vi "PSRR.vi"() -> ()   [LabVIEW 2020]
doc: "For every time interval of n second, where n is the Wait Time in seconds (not less than 2 seconds), the VI will call Synchronous PSRR.vi. If there are no errors, the obtained data will be plotted in a chart.\n\n1. Error Log - If Error Log is enabled, log entry into the Error Log Table (for both error and warning).\n2. Last Error Details – will be updated with the details of Last Error or Warning that happened.\n3. Error? - In case of an error, Error? LED will be ON until the error is cleared."
uses:
  Typedef/QueueOperation.ctl
  Typedef/State & Varaint.ctl
  Typedef/LV2_User_Event.ctl
  Typedef/Data Cluster.ctl
  Typedef/Timer_Cluster.ctl
  Typedef/LED_Colour.ctl
  <vilib>/Utility/miscctls.llb/LVRowAndColumnUnsignedTypeDef.ctl
panel:
  out "Error?":bool
  in  "Error Log":bool
  out "Error Log Table":string[][](table)
  in  "Exit":bool
  out "Time":string
  in  "Wait Time (sec)":i32=2 min=2
  out "Waveform Chart":i32(graph)
  out "Error Code":string
  out "Type":string
  out "Description":string
  out "Error Out":errorcluster
  out "Last Read PSRR (dB)":i32
  in  "Error In":errorcluster
  # "PSRR"
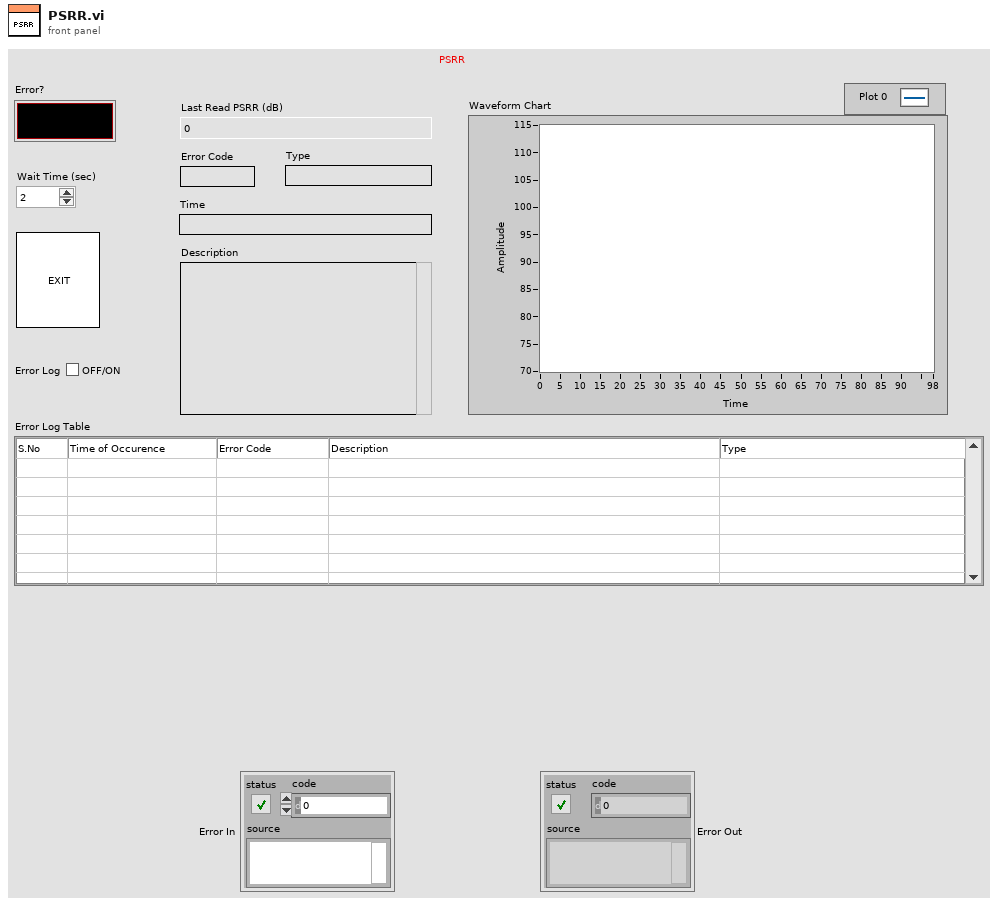
[diagram p1: front panel]
types:
  T1 = typedef "QueueOperation.ctl" = enum16{"Create", "Enqueue 1", "Enqueue N", "Enstack 1", "Enstack N", "Dequeue", "Flush", "Release"}
  T2 = typedef "LV2_User_Event.ctl" = enum16{"Create", "Generate", "Read", "Destroy"}
  T3 = typedef "State & Varaint.ctl" = cluster{"State":string, "Variant":variant}
  T4 = typedef "LVRowAndColumnUnsignedTypeDef.ctl" = cluster{"Row":u32, "Column":u32}
  T5 = typedef "Data Cluster.ctl" = cluster{"Exit":bool, "Error Log":bool, "Wait Time (sec)":i32, "Last Read PSRR (dB)":i32, "Waveform Chart":i32, "Error Code":string, "Type":string, "Time":string, "Description":string, "Error?":bool, "Error Info":errorcluster, "Timer":T6, "Passive Error Counter":i32, "Unknown Error Counter":i32, "Serial Number":i32, "Error Logging string array":string[][], "Popup Message":string, "Autoscroll":u32, "LED cluster":T7}
  T6 = typedef "Timer_Cluster.ctl" = cluster{"Previous":dbl, "Set Time":dbl, "Start":bool, "Elapsed":dbl}
  T7 = typedef "LED_Colour.ctl" = cluster{"Boolean Text":string, "Colors":cluster{u32, u32}[], "Txt Color":u32}
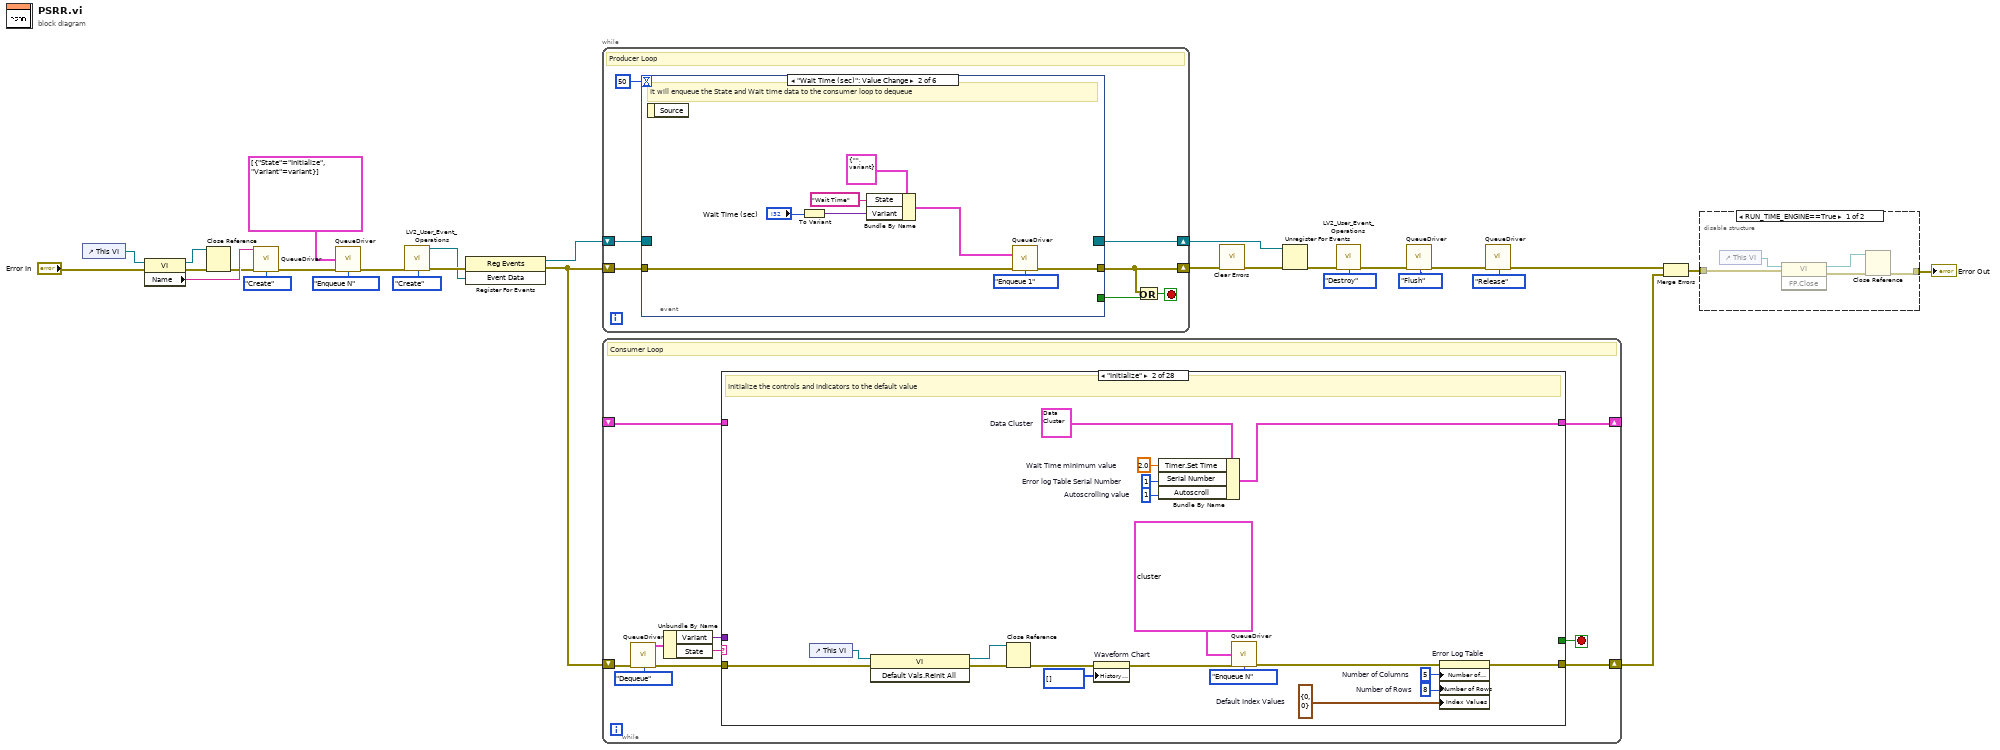
[diagram p0: block diagram]
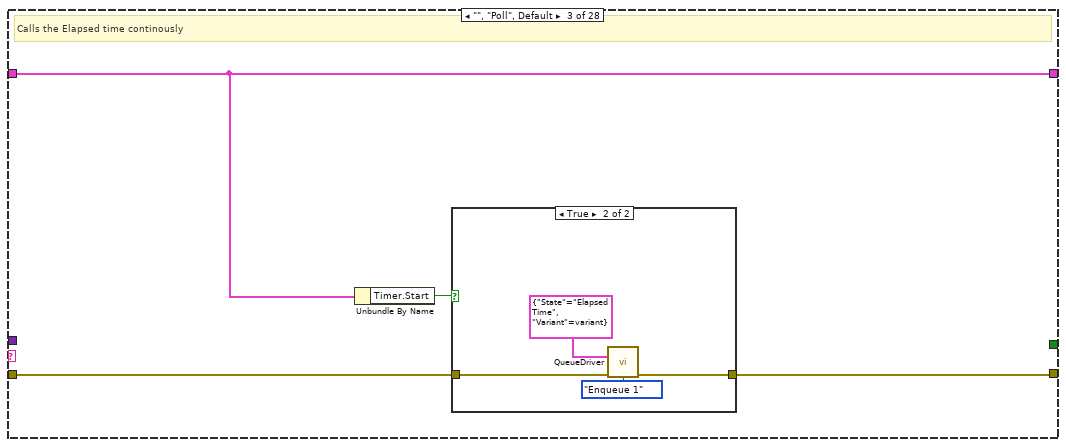
[diagram p4: hidden frame]
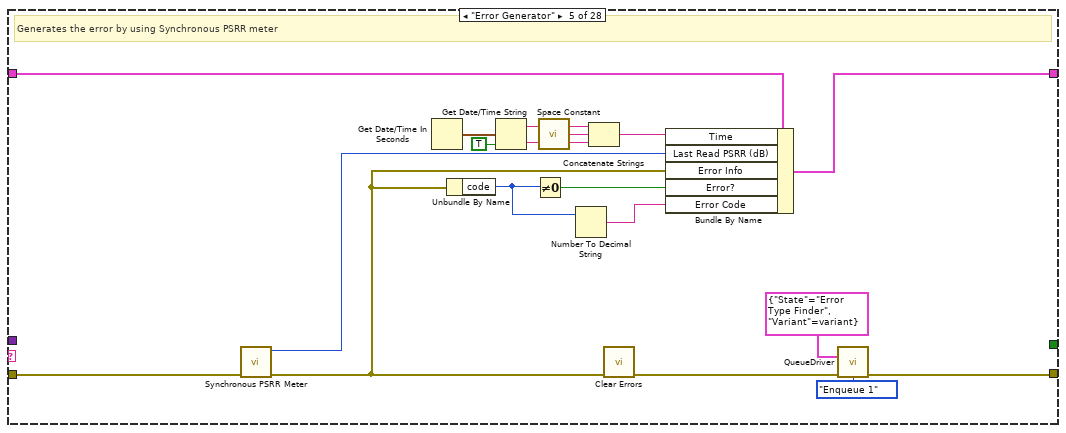
[diagram p7: hidden frame]
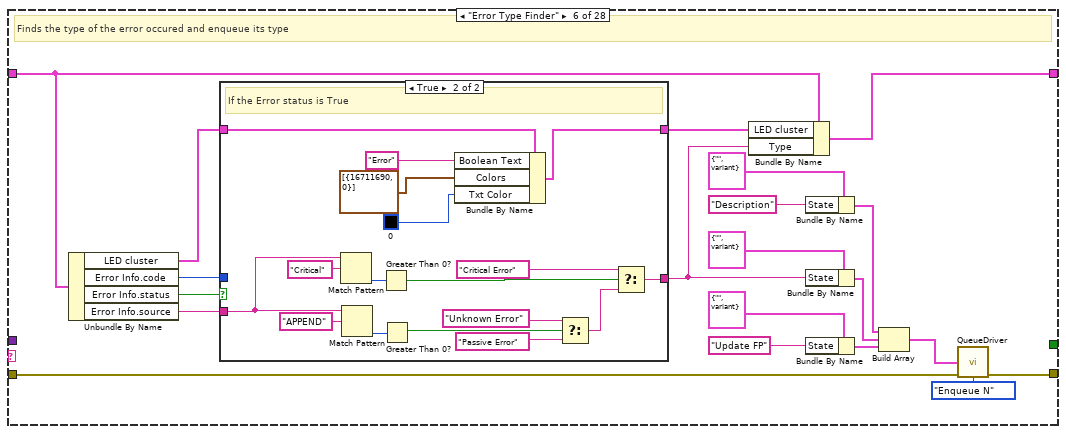
[diagram p8: hidden frame]
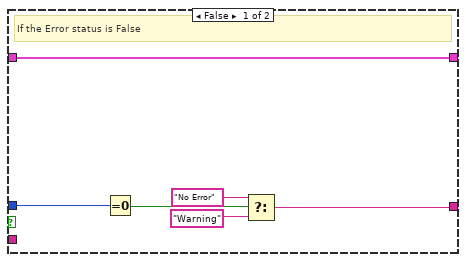
[diagram p9: hidden frame]
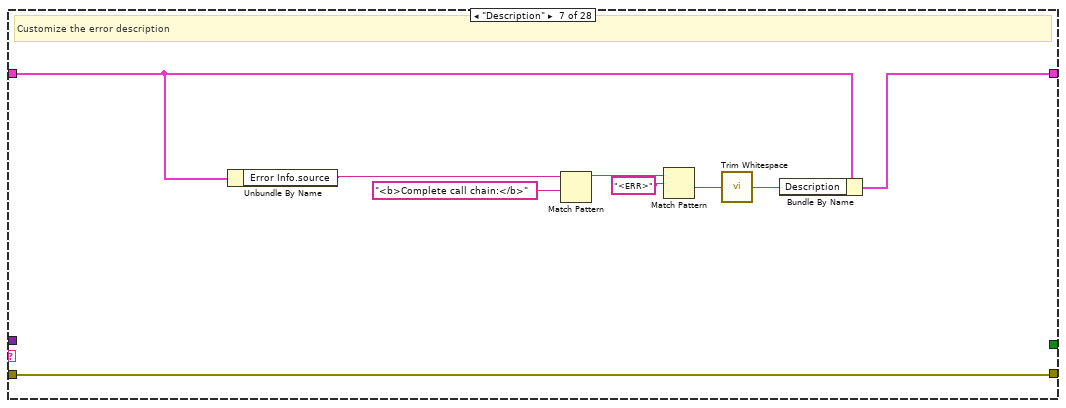
[diagram p10: hidden frame]
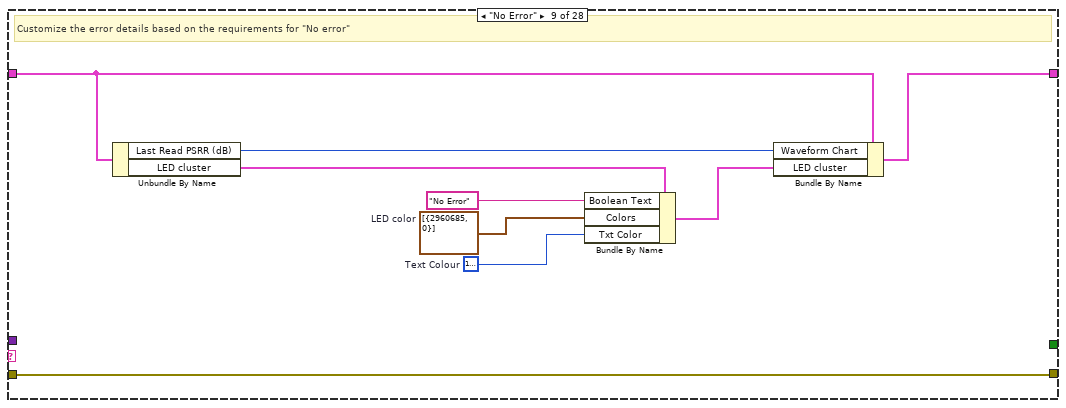
[diagram p12: hidden frame]
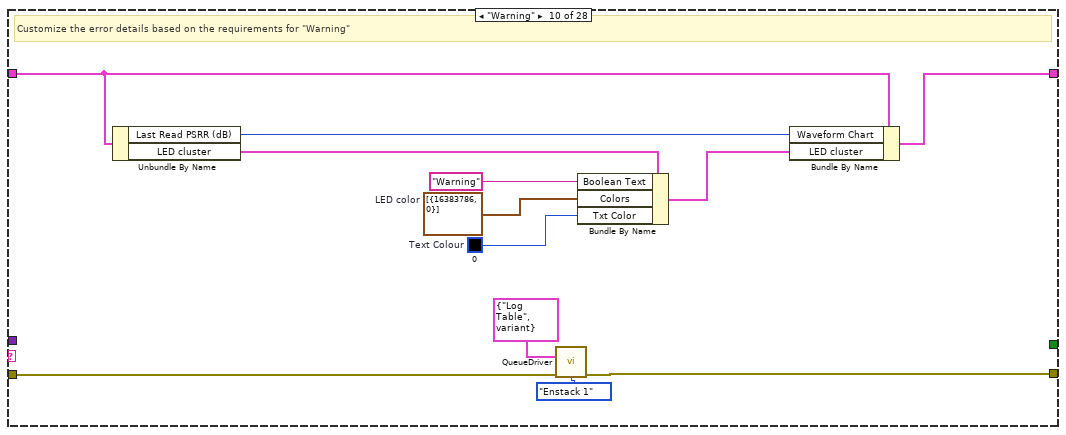
[diagram p13: hidden frame]
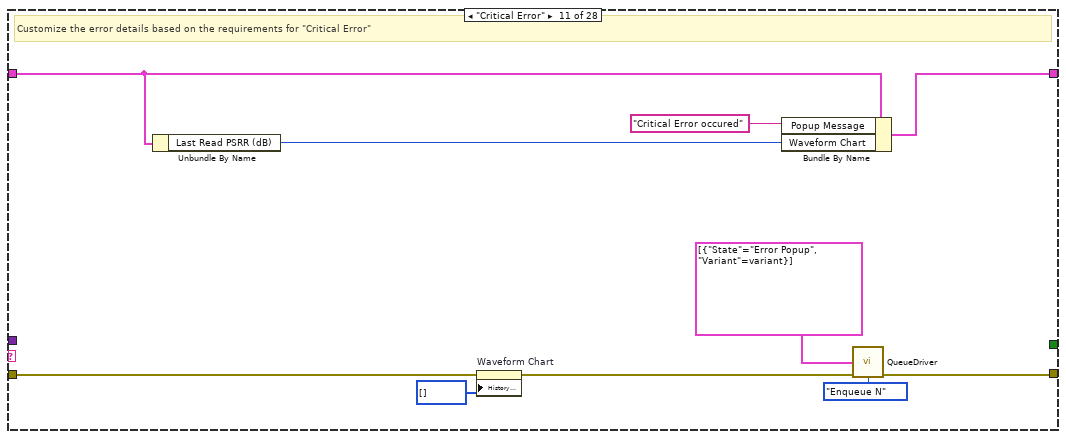
[diagram p14: hidden frame]
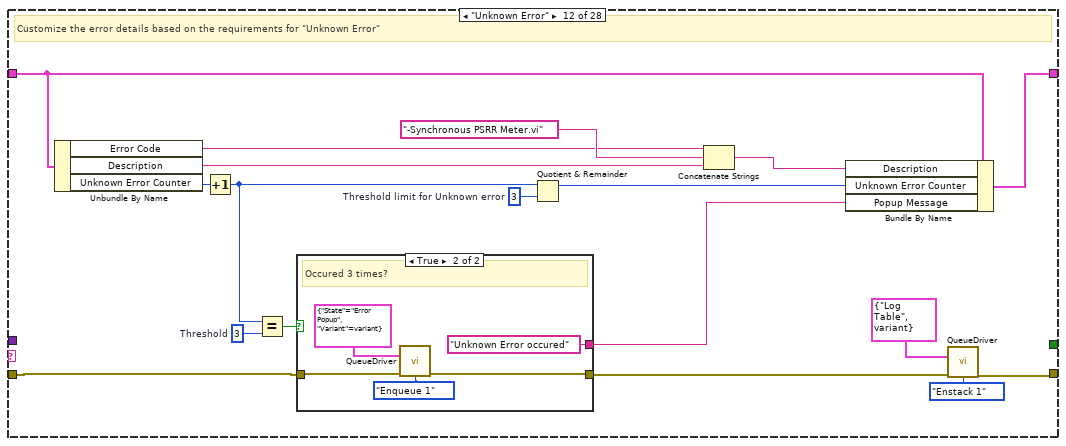
[diagram p15: hidden frame]
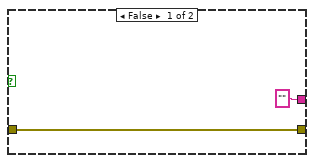
[diagram p16: hidden frame]
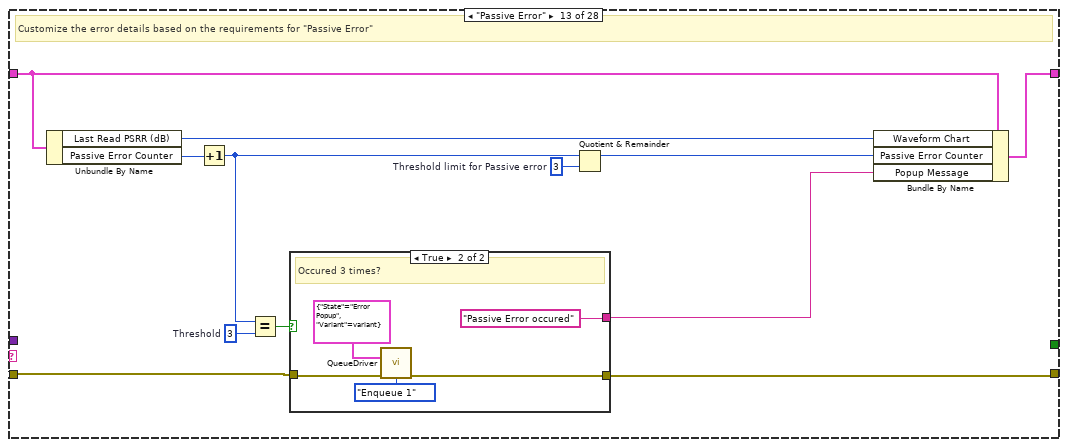
[diagram p17: hidden frame]
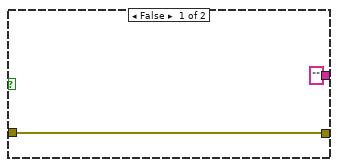
[diagram p18: hidden frame]
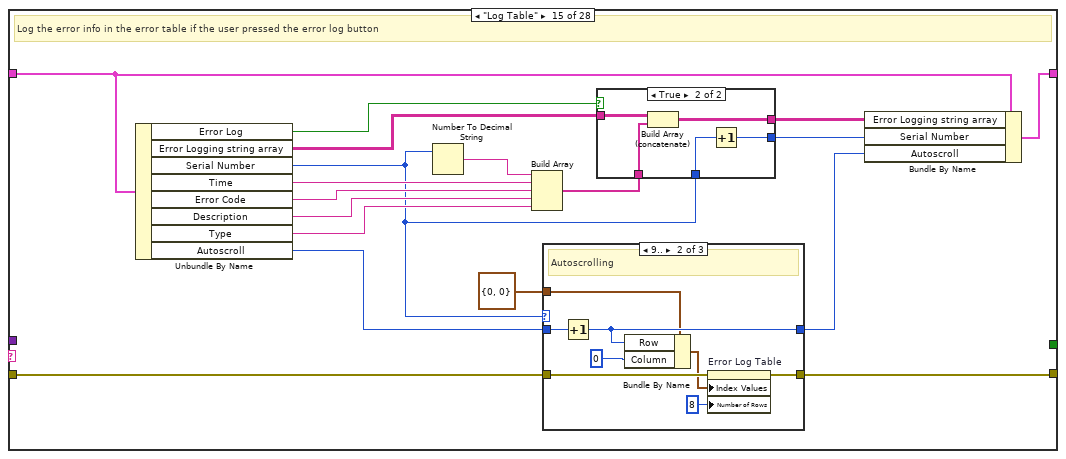
[diagram p20: hidden frame]
diagram:
  n1 = control-ref of="This VI"() -> (w6:refnum<vi>)
  n2 = property class="VI"(reference=w6, error in="Error In") -> (reference out=w3:refnum<vi>, error out=w5:errorcluster, "Name"=w27:string)
  n3 = Close Reference(reference=w3, error in (no error)=w5) -> (error out=w4:errorcluster)
  n4 = call "QueueDriver.vi"("Queue Name"=w27, "Error in (no error)"=w4, "Operations"=QueueOperation."Create") -> ("Error out"=w26:errorcluster)  [unwired: 11 in, 1 out]
  n5 = call "QueueDriver.vi"("Array of States & Data"=T3[] [{"State"="Initialize", "Variant"=variant}], "Error in (no error)"=w26, "Operations"=QueueOperation."Enqueue N") -> ("Error out"=w23:errorcluster)  [unwired: 11 in, 1 out]
  n6 = call "LV2_User_Event_Operations.vi"("Error In"=w23, "Operation"=LV2_User_Event."Create") -> ("Event Data"=w19:refnum<user-event>, "Error Out"=w21:errorcluster)  [unwired: 12 in]
  n7 = register-events(error in=w21, w19) -> (reference out=w18:refnum<event-registration>, error out=w20:errorcluster)  [unwired: 1 in]
  n8 = while {
    shift-right: [w30] -> w16
    shift-left: w20 -> [w35]
    shift-right: [w33] -> w14
    shift-left: w18 -> [w34]
    stop <- w32 stop-if-true
    # "Producer Loop"
    n9 = event shown="[1] \"Wait Time (sec)\": Value Change" {
      selector: w34 -> [_ _ _ _ _ _]
      dyn-events: [_ _ _ _ _ _] -> w33
      timeout: 50 -> [_ _ _ _ _ _]
      tunnel: [w37 w38 w52 w54 w58 w64] -> w30
      tunnel: w35 -> [w37 w45 w53 w54 w59 w65]
      tunnel: [_ _ _ TRUE w60 TRUE] -> w31
      event Timeout {
        # "This block executes when there is no event triggered"
        n10 = event-data() -> ()  [unwired: 1 in, 1 out]
      }
      event "Wait Time (sec)": Value Change {
        # "It will enqueue the State and Wait time data to the consumer loop to dequeue"
        n11 = event-data() -> ()  [unwired: 1 in, 1 out]
        n12 = To Variant(anything="Wait Time (sec)") -> (Variant=w40:variant)
        n13 = Bundle By Name(cluster=T3 {"State"="", "Variant"=variant} ("State & Data"), "State"="Wait Time", "Variant"=w40) -> (w39:T3)
        n14 = call "QueueDriver.vi"("State & Data"=w39, "Error in (no error)"=w45, "Operations"=QueueOperation."Enqueue 1") -> ("Error out"=w38:errorcluster)  [unwired: 11 in, 1 out]
      }
      event "Error Log": Value Change {
        # "It will enqueue the State and Error Log data to the consumer loop to dequeue"
        n15 = event-data() -> ()  [unwired: 1 in, 1 out]
        n16 = To Variant(anything="Error Log") -> (Variant=w48:variant)
        n17 = Bundle By Name(cluster=T3 {"State"="", "Variant"=variant} ("State & Data"), "State"="Error Log", "Variant"=w48) -> (w47:T3)
        n18 = call "QueueDriver.vi"("State & Data"=w47, "Error in (no error)"=w53, "Operations"=QueueOperation."Enqueue 1") -> ("Error out"=w52:errorcluster)  [unwired: 11 in, 1 out]
      }
      event User Event {
        # "Stops the producer loop when consumer loop generates the user event"
        n19 = event-data() -> ()  [unwired: 1 in, 1 out]
      }
      event Panel Close? {
        w60 = TRUE
        # "Stops the VI when the panel close button is pressed"
        n20 = event-data() -> ()  [unwired: 1 in, 1 out]
        n21 = call "QueueDriver.vi"("State & Data"=T3 {"State"="Exit", "Variant"=variant}, "Error in (no error)"=w59, "Operations"=QueueOperation."Enstack 1") -> ("Error out"=w58:errorcluster)  [unwired: 11 in, 1 out]
        n22 = event-data("Discard?"=w60) -> ()  [unwired: 1 in, 1 out]
      }
      event "Exit": Value Change {
        # "Stops the VI when the exit button is pressed"
        n23 = event-data() -> ()  [unwired: 1 in, 1 out]
        n24 = call "QueueDriver.vi"("State & Data"=T3 {"State"="Exit", "Variant"=variant}, "Error in (no error)"=w65, "Operations"=QueueOperation."Enstack 1") -> ("Error out"=w64:errorcluster)  [unwired: 11 in, 1 out]
      }
    }
    n25 = Or(x=w30, y=w31) -> (x .or. y?=w32:bool)
  }
  n26 = while {
    shift-right: [w69] -> w13
    shift-left: w20 -> [w75]
    shift-right: [w68] -> _
    shift-left: _ -> [w67]
    stop <- w66 stop-if-true
    # "Consumer Loop"
    n27 = call "QueueDriver.vi"("Error in (no error)"=w75, "Operations"=QueueOperation."Dequeue") -> ("Dequeued State & Variant"=w73:T3, "Error out"=w70:errorcluster)  [unwired: 12 in]
    n28 = Unbundle By Name(w73) -> ("Variant"=w71:variant, "State"=w72:string)
    n29 = case shown="\"Initialize\"" w72 {
      tunnel: w71 -> [_ _ _ _ _ _ _ _ _ _ _ _ _ _ _ _ _ _ w337 w345 _ _ _ _ _ _ _ _]
      tunnel: w70 -> [w76 w96 w100 w107 w125 w142 w169 w179 w185 w196 w202 w215 w236 w256 w263 w304 w318 w332 w339 w346 w348 w350 w359 w371 w379 w384 w400 w401]
      tunnel: [w76 w84 w99 w107 w121 w141 w169 w179 w185 w197 w206 w225 w238 w256 w264 w305 w317 w332 w334 w343 w348 w350 w359 w370 w379 w381 w400 w404] -> w69
      tunnel: [w77 w92 w97 w106 w123 w143 w176 w178 w187 w199 w209 w226 w246 w255 w273 w307 w322 w331 w333 w342 w347 w354 w358 w368 w378 w383 w399 w405] -> w68
      tunnel: w67 -> [w77 _ w97 w106 w124 w144 w177 w178 w188 w200 w210 w228 w247 w255 w274 w307 w322 w331 w336 w344 w347 w355 w360 w369 w378 w383 w399 w405]
      tunnel: [_ _ _ _ _ _ _ _ _ _ _ _ _ _ _ _ _ _ _ _ _ _ _ _ _ w380 _ TRUE] -> w66
      frame "/*******Initialize the VI*******/" {
      }
      frame "Initialize" {
        w81 = T4 {"Row"=0, "Column"=0}  # Default Index Values
        w82 = u32 8  # Number of Rows
        w83 = u32 5  # Number of Columns
        w86 = u32 1  # Autoscrolling value
        w90 = 1  # Error log Table Serial Number
        w91 = 2.0  # Wait Time minimum value
        w94 = T5 {"Exit"=FALSE, "Error Log"=FALSE, "Wait Time (sec)"=0, "Last Read PSRR (dB)"=0, "Waveform Chart"=0, "Error Code"="", "Type"="", "Time"="", "Description"="", "Error?"=FALSE, "Error Info"={"status"=FALSE, "code"=0, "source"=""}, "Timer"={"Previous"=0.0, "Set Time"=0.0, "Start"=FALSE, "Elapsed"=0.0}, "Passive Error Counter"=0, "Unknown Error Counter"=0, "Serial Number"=0, "Error Logging string array"=[], "Popup Message"="", "Autoscroll"=0, "LED cluster"={"Boolean Text"="", "Colors"=[], "Txt Color"=0}}  # Data Cluster
        # "Initialize the controls and indicators to the default value"
        n30 = control-ref of="This VI"() -> (w88:refnum<vi>)
        n31 = invoke class="VI" method="Default Vals.Reinit All"(reference=w88, error in=w96) -> (reference out=w87:refnum<vi>, error out=w89:errorcluster)  [unwired: 1 in, 1 out]
        n32 = Close Reference(reference=w87, error in (no error)=w89) -> (error out=w79:errorcluster)
        n33 = property on="Waveform Chart" class="WFChart (strict)"(error in=w79, "History Data"=i32[] []) -> (error out=w78:errorcluster)  [unwired: 1 in, 1 out]
        n34 = Bundle By Name(cluster=w94, "Timer.Set Time"=w91, "Serial Number"=w90, "Autoscroll"=w86) -> (w92:T5)
        n35 = call "QueueDriver.vi"("Array of States & Data"=T3[] [{"State"="Start", "Variant"=variant}, {"State"="Error Generator", "Variant"=variant}], "Error in (no error)"=w78, "Operations"=QueueOperation."Enqueue N") -> ("Error out"=w85:errorcluster)  [unwired: 11 in, 1 out]
        n36 = property on="Error Log Table" class="Tbl (strict)"(error in=w85, "Number of Columns"=w83, "Number of Rows"=w82, "Index Values"=w81) -> (error out=w84:errorcluster)  [unwired: 1 in, 1 out]
      }
      frame "", "Poll", Default {
        # "Calls the Elapsed time continously"
        n37 = Unbundle By Name(w97) -> ("Timer.Start"=w98:bool)
        n38 = case shown="True" w98 {
          tunnel: w100 -> [w101 w105]
          tunnel: [w101 w102] -> w99
          frame False {
          }
          frame True {
            n39 = call "QueueDriver.vi"("State & Data"=T3 {"State"="Elapsed Time", "Variant"=variant}, "Error in (no error)"=w105, "Operations"=QueueOperation."Enqueue 1") -> ("Error out"=w102:errorcluster)  [unwired: 11 in, 1 out]
          }
        }
      }
      frame "/*******Error Generation*******/" {
      }
      frame "Error Generator" {
        # "Generates the error by using Synchronous PSRR meter"
        n40 = call "Synchronous PSRR Meter.vi"("error in"=w125) -> ("error out"=w112:errorcluster, "PSRR (dB)"=w113:i32)  [unwired: 9 in]
        n41 = Get Date/Time In Seconds() -> (seconds since 1Jan1904=w118:timestamp)
        n42 = Unbundle By Name(w112) -> ("code"=w110:i32)
        n43 = Get Date/Time String(seconds (now)=w118, want seconds? (F)=TRUE) -> (date string=w117:string, time string=w115:string)  [unwired: 1 in]
        n44 = Not Equal To 0?(x=w110) -> (x != 0?=w111:bool)
        n45 = call <vilib>:"Space Constant.vi"() -> ("String"=w114:string)
        n46 = Number To Decimal String(number=w110) -> (decimal integer string=w109:string)  [unwired: 1 in]
        n47 = Concatenate Strings(w117, w114, w115) -> (w108:string)
        n48 = call <vilib>:"Clear Errors.vi"("error in (no error)"=w112) -> ("error out"=w122:errorcluster)  [unwired: 5 in, 1 out]
        n49 = Bundle By Name(cluster=w124, "Time"=w108, "Last Read PSRR (dB)"=w113, "Error Info"=w112, "Error?"=w111, "Error Code"=w109) -> (w123:T5)
        n50 = call "QueueDriver.vi"("State & Data"=T3 {"State"="Error Type Finder", "Variant"=variant}, "Error in (no error)"=w122, "Operations"=QueueOperation."Enqueue 1") -> ("Error out"=w121:errorcluster)  [unwired: 11 in, 1 out]
      }
      frame "Error Type Finder" {
        # "Finds the type of the error occured and enqueue its type"
        n51 = Unbundle By Name(w144) -> ("LED cluster"=w126:T7, "Error Info.code"=w134:i32, "Error Info.status"=w145:bool, "Error Info.source"=w139:string)
        n52 = case shown="True" w145 {
          tunnel: w139 -> [_ w157]
          tunnel: [w148 w158] -> w130
          tunnel: w134 -> [w147 _]
          tunnel: [w146 w153] -> w127
          tunnel: w126 -> [w146 w152]
          frame False {
            # "If the Error status is False"
            n53 = Equal To 0?(x=w147) -> (x = 0?=w151:bool)
            n54 = Select(t="No Error" ("regular expression"), s=w151, f="Warning" ("regular expression")) -> (s? t:f=w148:string)
          }
          frame True {
            # "If the Error status is True"
            n55 = Match Pattern(string=w157, regular expression="Critical") -> (offset past match=w167:i32)  [unwired: 1 in, 3 out]
            n56 = Match Pattern(string=w157, regular expression="APPEND") -> (offset past match=w164:i32)  [unwired: 1 in, 3 out]
            n57 = Greater Than 0?(x=w167) -> (x > 0?=w166:bool)
            n58 = Greater Than 0?(x=w164) -> (x > 0?=w163:bool)
            n59 = Bundle By Name(cluster=w152, "Boolean Text"="Error" ("Boolean Text.Text"), "Colors"=cluster{u32, u32}[] [{16711690, 0}] ("Colors [4]"), "Txt Color"=u32 0) -> (w153:T7)
            n60 = Select(t="Unknown Error" ("regular expression"), s=w163, f="Passive Error") -> (s? t:f=w159:string)
            n61 = Select(t="Critical Error" ("regular expression"), s=w166, f=w159) -> (s? t:f=w158:string)
          }
        }
        n62 = Bundle By Name(cluster=w144, "LED cluster"=w127, "Type"=w130) -> (w143:T5)
        n63 = Bundle By Name(cluster=T3 {"State"="", "Variant"=variant} ("State & Data"), "State"="Description") -> (w133:T3)
        n64 = Bundle By Name(cluster=T3 {"State"="", "Variant"=variant} ("State & Data"), "State"=w130) -> (w136:T3)
        n65 = Bundle By Name(cluster=T3 {"State"="", "Variant"=variant} ("State & Data"), "State"="Update FP") -> (w137:T3)
        n66 = Build Array(w133, w136, w137) -> (w135:T3[])
        n67 = call "QueueDriver.vi"("Array of States & Data"=w135, "Error in (no error)"=w142, "Operations"=QueueOperation."Enqueue N") -> ("Error out"=w141:errorcluster)  [unwired: 11 in, 1 out]
      }
      frame "Description" {
        # "Customize the error description"
        n68 = Unbundle By Name(w177) -> ("Error Info.source"=w171:string)
        n69 = Match Pattern(string=w171, regular expression="<b>Complete call chain:</b>") -> (before substring=w174:string)  [unwired: 1 in, 3 out]
        n70 = Match Pattern(string=w174, regular expression="<ERR>") -> (after substring=w172:string)  [unwired: 1 in, 3 out]
        n71 = call <vilib>:"Trim Whitespace.vi"("string"=w172) -> ("trimmed string"=w170:string)  [unwired: 1 in]
        n72 = Bundle By Name(cluster=w177, "Description"=w170) -> (w176:T5)
      }
      frame "/*******Error Handling*******/" {
      }
      frame "No Error" {
        w182 = u32 16777225  # Text Colour
        w183 = cluster{u32, u32}[] [{2960685, 0}]  # LED color
        # "Customize the error details based on the requirements for \"No error\""
        n73 = Unbundle By Name(w188) -> ("Last Read PSRR (dB)"=w186:i32, "LED cluster"=w180:T7)
        n74 = Bundle By Name(cluster=w180, "Boolean Text"="No Error" ("Boolean Text.Text"), "Colors"=w183, "Txt Color"=w182) -> (w181:T7)
        n75 = Bundle By Name(cluster=w188, "Waveform Chart"=w186, "LED cluster"=w181) -> (w187:T5)
      }
      frame "Warning" {
        w191 = u32 0  # Text Colour
        w192 = cluster{u32, u32}[] [{16383786, 0}]  # LED color
        # "Customize the error details based on the requirements for \"Warning\""
        n76 = Unbundle By Name(w200) -> ("Last Read PSRR (dB)"=w198:i32, "LED cluster"=w189:T7)
        n77 = call "QueueDriver.vi"("State & Data"=T3 {"State"="Log Table", "Variant"=variant}, "Error in (no error)"=w196, "Operations"=QueueOperation."Enstack 1") -> ("Error out"=w197:errorcluster)  [unwired: 11 in, 1 out]
        n78 = Bundle By Name(cluster=w189, "Boolean Text"="Warning" ("Boolean Text.Text"), "Colors"=w192, "Txt Color"=w191) -> (w190:T7)
        n79 = Bundle By Name(cluster=w200, "Waveform Chart"=w198, "LED cluster"=w190) -> (w199:T5)
      }
      frame "Critical Error" {
        # "Customize the error details based on the requirements for \"Critical Error\""
        n80 = Unbundle By Name(w210) -> ("Last Read PSRR (dB)"=w208:i32)
        n81 = property on="Waveform Chart" class="WFChart (strict)"(error in=w202, "History Data"=i32[] []) -> (error out=w203:errorcluster)  [unwired: 1 in, 1 out]
        n82 = Bundle By Name(cluster=w210, "Popup Message"="Critical Error occured" ("message"), "Waveform Chart"=w208) -> (w209:T5)
        n83 = call "QueueDriver.vi"("Array of States & Data"=T3[] [{"State"="Error Popup", "Variant"=variant}], "Error in (no error)"=w203, "Operations"=QueueOperation."Enqueue N") -> ("Error out"=w206:errorcluster)  [unwired: 11 in, 1 out]
      }
      frame "Unknown Error" {
        w217 = 3  # Threshold limit for Unknown error
        w220 = 3  # Threshold
        # "Customize the error details based on the requirements for \"Unknown Error\""
        n84 = Unbundle By Name(w228) -> ("Error Code"=w211:string, "Description"=w227:string, "Unknown Error Counter"=w221:i32)
        n85 = Increment(x=w221) -> (x+1=w218:i32)
        n86 = Equal?(x=w218, y=w220) -> (x = y?=w219:bool)
        n87 = case shown="True" w219 {
          tunnel: w215 -> [w230 w232]
          tunnel: [w230 w234] -> w222
          tunnel: ["" ("message") "Unknown Error occured" ("message")] -> w214
          frame False {
          }
          frame True {
            # "Occured 3 times?"
            n88 = call "QueueDriver.vi"("State & Data"=T3 {"State"="Error Popup", "Variant"=variant}, "Error in (no error)"=w232, "Operations"=QueueOperation."Enqueue 1") -> ("Error out"=w234:errorcluster)  [unwired: 11 in, 1 out]
          }
        }
        n89 = Quotient & Remainder(x=w218, y=w217) -> (x-y*floor(x/y)=w216:i32)  [unwired: 1 out]
        n90 = Concatenate Strings(w211, "-Synchronous PSRR Meter.vi" ("string"), w227) -> (w223:string)
        n91 = Bundle By Name(cluster=w228, "Description"=w223, "Unknown Error Counter"=w216, "Popup Message"=w214) -> (w226:T5)
        n92 = call "QueueDriver.vi"("State & Data"=T3 {"State"="Log Table", "Variant"=variant}, "Error in (no error)"=w222, "Operations"=QueueOperation."Enstack 1") -> ("Error out"=w225:errorcluster)  [unwired: 11 in, 1 out]
      }
      frame "Passive Error" {
        w240 = 3  # Threshold limit for Passive error
        w243 = 3  # Threshold
        # "Customize the error details based on the requirements for \"Passive Error\""
        n93 = Unbundle By Name(w247) -> ("Last Read PSRR (dB)"=w245:i32, "Passive Error Counter"=w244:i32)
        n94 = Increment(x=w244) -> (x+1=w241:i32)
        n95 = Equal?(x=w241, y=w243) -> (x = y?=w242:bool)
        n96 = case shown="True" w242 {
          tunnel: w236 -> [w248 w252]
          tunnel: [w248 w251] -> w238
          tunnel: ["" ("message") "Passive Error occured" ("message")] -> w237
          frame False {
          }
          frame True {
            # "Occured 3 times?"
            n97 = call "QueueDriver.vi"("State & Data"=T3 {"State"="Error Popup", "Variant"=variant}, "Error in (no error)"=w252, "Operations"=QueueOperation."Enqueue 1") -> ("Error out"=w251:errorcluster)  [unwired: 11 in, 1 out]
          }
        }
        n98 = Quotient & Remainder(x=w241, y=w240) -> (x-y*floor(x/y)=w239:i32)  [unwired: 1 out]
        n99 = Bundle By Name(cluster=w247, "Waveform Chart"=w245, "Passive Error Counter"=w239, "Popup Message"=w237) -> (w246:T5)
      }
      frame "/*******User Interface*******/" {
      }
      frame "Log Table" {
        # "Log the error info in the error table if the user pressed the error log button"
        n100 = Unbundle By Name(w274) -> ("Error Log"=w260:bool, "Error Logging string array"=w272:string[][], "Serial Number"=w258:i32, "Time"=w270:string, "Error Code"=w269:string, "Description"=w268:string, "Type"=w267:string, "Autoscroll"=w262:u32)
        n101 = Number To Decimal String(number=w258) -> (decimal integer string=w271:string)  [unwired: 1 in]
        n102 = Build Array(w271, w270, w269, w268, w267) -> (w265:string[])
        n103 = case shown="9.." w258 {
          tunnel: [w283 w291 w299] -> w264
          tunnel: w263 -> [w283 w290 w298]
          tunnel: w262 -> [w282 w286 w294]
          tunnel: [w282 w285 w294] -> w261
          tunnel: T4 {"Row"=0, "Column"=0} ("Index Values") -> [_ w284 w292]
          frame 0, Default {
            # "No Autoscrolling"
          }
          frame 9.. {
            # "Autoscrolling"
            n104 = Increment(x=w286) -> (x+1=w285:u32)
            n105 = Bundle By Name(cluster=w284, "Row"=w285, "Column"=u32 0) -> (w288:T4)
            n106 = property on="Error Log Table" class="Tbl (strict)"(error in=w290, "Index Values"=w288, "Number of Rows"=u32 8) -> (error out=w291:errorcluster)  [unwired: 1 in, 1 out]
          }
          frame 8 {
            # "Autoscrolling"
            n107 = Bundle By Name(cluster=w292, "Row"=u32 1, "Column"=u32 0) -> (w296:T4)
            n108 = property on="Error Log Table" class="Tbl (strict)"(error in=w298, "Index Values"=w296, "Number of Rows"=u32 8) -> (error out=w299:errorcluster)  [unwired: 1 in, 1 out]
          }
        }
        n109 = case shown="True" w260 {
          tunnel: w272 -> [w276 w281]
          tunnel: [w276 w280] -> w266
          tunnel: w265 -> [_ w279]
          tunnel: [w275 w278] -> w259
          tunnel: w258 -> [w275 w277]
          frame False {
          }
          frame True {
            n110 = Build Array (concatenate)(w281, w279) -> (w280:string[][])
            n111 = Increment(x=w277) -> (x+1=w278:i32)
          }
        }
        n112 = Bundle By Name(cluster=w274, "Error Logging string array"=w266, "Serial Number"=w259, "Autoscroll"=w261) -> (w273:T5)
      }
      frame "Update FP" {
        # "Updates the Front Panel"
        n113 = Unbundle By Name(w307) -> ("Last Read PSRR (dB)"=→"Last Read PSRR (dB)":i32, "Waveform Chart"=→"Waveform Chart":i32, "Error Code"=→"Error Code":string, "Type"=→"Type":string, "Time"=→"Time":string, "Description"=→"Description":string, "Error Logging string array"=→"Error Log Table":string[][], "Error?"=→"Error?":bool, "LED cluster"=w303:T7)
        n114 = Unbundle By Name(w303) -> ("Boolean Text"=w302:string, "Colors"=w301:cluster{u32, u32}[], "Txt Color"=w300:u32)
        n115 = property on="Error?" class="Bool (strict)"(error in=w304, "BoolText.Text"=w302, "Colors [4]"=w301, "BoolText.TextColor"=w300) -> (error out=w305:errorcluster)  [unwired: 1 in, 1 out]
      }
      frame "Error Popup" {
        # "If error occurs, It will raise the popup"
        n116 = Unbundle By Name(w322) -> ("Popup Message"=w321:string)
        n117 = Two Button Dialog(message=w321, 1:"Stop" ("F button name (\"Cancel\")"), 2:"Continue" ("T button name (\"OK\")")) -> (T button?=w316:bool)
        n118 = Not(x=w316) -> (.not. x?=w315:bool)
        n119 = case shown="False" w315 {
          tunnel: w318 -> [w323 w330]
          tunnel: [w324 w329] -> w317
          frame False {
            # "Resume the time"
            n120 = call "QueueDriver.vi"("State & Data"=T3 {"State"="Resume", "Variant"=variant}, "Error in (no error)"=w323, "Operations"=QueueOperation."Enstack 1") -> ("Error out"=w324:errorcluster)  [unwired: 11 in, 1 out]
          }
          frame True {
            # "Stops the VI"
            n121 = call "QueueDriver.vi"("State & Data"=T3 {"State"="Exit", "Variant"=variant}, "Error in (no error)"=w330, "Operations"=QueueOperation."Enstack 1") -> ("Error out"=w329:errorcluster)  [unwired: 11 in, 1 out]
          }
        }
      }
      frame "/*******Read Data*******/" {
      }
      frame "Wait Time" {
        # "Reads the wait time data from Producer"
        n122 = Variant To Data(error in=w339, type=0.0 ("Wait Time (sec)"), Variant=w337) -> (data=w335:dbl, error out=w334:errorcluster)
        n123 = Bundle By Name(cluster=w336, "Timer.Set Time"=w335) -> (w333:T5)
      }
      frame "Error Log" {
        # "Reads the error log data from Producer"
        n124 = Variant To Data(error in=w346, type=FALSE, Variant=w345) -> (data=w340:bool, error out=w343:errorcluster)
        n125 = Bundle By Name(cluster=w344, "Error Log"=w340) -> (w342:T5)
      }
      frame "/*******Timer*******/" {
      }
      frame "Start" {
        # "Starts the timer to generate the error"
        n126 = Get Date/Time In Seconds() -> (seconds since 1Jan1904=w352:timestamp)
        n127 = To Double Precision Float(number=w352) -> (double precision float=w351:dbl)
        n128 = Bundle By Name(cluster=w355, "Timer.Start"=TRUE, "Timer.Previous"=w351, "Timer.Elapsed"=0.0) -> (w354:T5)
      }
      frame "Resume" {
        # "Updates the current time after closing the error popup"
        n129 = Get Date/Time In Seconds() -> (seconds since 1Jan1904=w357:timestamp)
        n130 = To Double Precision Float(number=w357) -> (double precision float=w356:dbl)
        n131 = Bundle By Name(cluster=w360, "Timer.Previous"=w356) -> (w358:T5)
      }
      frame "Elapsed Time" {
        # "Calculates the elpased time and runs the PSRR meter"
        n132 = Unbundle By Name(w369) -> ("Timer.Previous"=w365:dbl, "Timer.Elapsed"=w363:dbl, "Timer.Set Time"=w367:dbl)
        n133 = Get Date/Time In Seconds() -> (seconds since 1Jan1904=w366:timestamp)
        n134 = To Double Precision Float(number=w366) -> (double precision float=w361:dbl)
        n135 = Subtract(x=w361, y=w365) -> (x-y=w364:dbl)
        n136 = Add(x=w364, y=w363) -> (x+y=w362:dbl)
        n137 = Less?(x=w362, y=w367) -> (x < y?=w372:bool)
        n138 = case shown="False" w372 {
          tunnel: w371 -> [w376 w377]
          tunnel: [w375 w377] -> w370
          frame False {
            # "It will generate the error using PSRR"
            n139 = call "QueueDriver.vi"("Array of States & Data"=T3[] [{"State"="Start", "Variant"=variant}, {"State"="Error Generator", "Variant"=variant}], "Error in (no error)"=w376, "Operations"=QueueOperation."Enqueue N") -> ("Error out"=w375:errorcluster)  [unwired: 11 in, 1 out]
          }
          frame True {
            # "Continue"
          }
        }
        n140 = Bundle By Name(cluster=w369, "Timer.Previous"=w361, "Timer.Elapsed"=w362) -> (w368:T5)
      }
      frame "/*******Error Case*******/" {
      }
      frame "Error" {
        # "If error has occured, It will raise the popup and asks user to whether continue the process or stop the VI."
        n141 = Unbundle By Name(w384) -> ("source"=w393:string, "code"=w391:i32)
        n142 = Number To Decimal String(number=w391) -> (decimal integer string=w389:string)  [unwired: 1 in]
        n143 = Concatenate Strings(w393, "\r\n", "Error Code : " ("string"), w389) -> (w388:string)
        n144 = Two Button Dialog(message=w388, 1:"Stop" ("F button name (\"Cancel\")"), 2:"Continue" ("T button name (\"OK\")")) -> (T button?=w385:bool)
        n145 = Not(x=w385) -> (.not. x?=w380:bool)
        n146 = call <vilib>:"Clear Errors.vi"("error in (no error)"=w384) -> ("error out"=w382:errorcluster)  [unwired: 5 in, 1 out]
        n147 = case shown="True" w380 {
          tunnel: w382 -> [w394 w397]
          tunnel: [w394 w396] -> w381
          frame False {
            # "Continue the process"
          }
          frame True {
            # "Stops the VI by using user event"
            n148 = call "LV2_User_Event_Operations.vi"("Event Data"=0.0, "Error In"=w397, "Operation"=LV2_User_Event."Generate") -> ("Error Out"=w396:errorcluster)  [unwired: 11 in, 1 out]
          }
        }
      }
      frame "/*******Stops the VI*******/" {
      }
      frame "Exit" {
        # "Stops the VI"
        n149 = call "LV2_User_Event_Operations.vi"("Event Data"=0.0, "Error In"=w401, "Operation"=LV2_User_Event."Generate") -> ("Error Out"=w404:errorcluster)  [unwired: 11 in, 1 out]
      }
    }
  }
  n150 = call <vilib>:"Clear Errors.vi"("error in (no error)"=w16) -> ("error out"=w7:errorcluster)  [unwired: 5 in, 1 out]
  n151 = Unregister For Events(event registration refnum=w14, error in=w7) -> (error out=w15:errorcluster)
  n152 = call "LV2_User_Event_Operations.vi"("Error In"=w15, "Operation"=LV2_User_Event."Destroy") -> ("Error Out"=w12:errorcluster)  [unwired: 12 in, 1 out]
  n153 = call "QueueDriver.vi"("Error in (no error)"=w12, "Operations"=QueueOperation."Flush") -> ("Error out"=w10:errorcluster)  [unwired: 12 in, 1 out]
  n154 = call "QueueDriver.vi"("Error in (no error)"=w10, "Operations"=QueueOperation."Release") -> ("Error out"=w9:errorcluster)  [unwired: 12 in, 1 out]
  n155 = Merge Errors(w9, w13) -> (w2:errorcluster)
  n156 = disable-structure shown="RUN_TIME_ENGINE==True" {
    disable-tunnel: w2 -> [w408 w412]
    disable-tunnel: [w407 w412] -> w1
    frame condition #0 {
      n157 = control-ref of="This VI"() -> (w410:refnum<vi>)
      n158 = invoke class="VI" method="FP.Close"(reference=w410, error in=w408) -> (reference out=w409:refnum<vi>, error out=w411:errorcluster)  [unwired: 1 in, 1 out]
      n159 = Close Reference(reference=w409, error in (no error)=w411) -> (error out=w407:errorcluster)
    }
    frame condition #1 (active) {
    }
  }
  "Error Out" <- w1
